vi "determinXY.vi"(0 "x max":dbl, 1 "x min":dbl, 2 "x":dbl, 3 "y max":dbl, 4 "y min":dbl, 5 "y":dbl) -> (6 "result":bool)   [LabVIEW 2014]
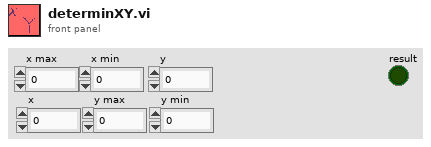
[diagram p1: front panel]
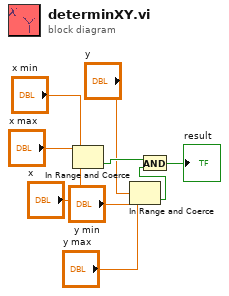
[diagram p0: block diagram]
diagram:
  n1 = In Range and Coerce(upper limit="x max", x="x", lower limit="x min") -> (In Range?=w9:bool)  [unwired: 1 out]
  n2 = In Range and Coerce(upper limit="y max", x="y", lower limit="y min") -> (In Range?=w8:bool)  [unwired: 1 out]
  n3 = And(x=w9, y=w8) -> (x .and. y?=→"result":bool)
